vi "LoadDocument__slk_msxml.vi"(0 "document in":refnum<class "msxml document.lvclass">, 1 "xml document path in":path, 11 "error in (no error)":errorcluster, 12 "validate on parse (F)":bool) -> (4 "document out":refnum<class "msxml document.lvclass">, 15 "error out":errorcluster)   [LabVIEW 2020, in "MSXML.lvlib" / "msxml document.lvclass"]
doc: "Loads an XML file to MSXML Document object and allows you to configure the XML parser to validate the file against a schema or DTD (Document Type Definition)."
uses:
  msxml document.lvclass
  msxml document.lvclass/msxml document.ctl
panel:
  # "LoadDocument__slk_msxml.vi\n\nLoads an XML file to MSXML Document object and allows you to configure the XML parser to validate the file against a schema or DTD (Document Type Definition).\n\nNOTICE -- YOU MUST LEAVE THIS NOTICE IN PLACE.\n\nCopyright (c) 2004-2010 Shawn Liu <shawn.liu.cn@gmail.com>\n\nAll rights reserved."
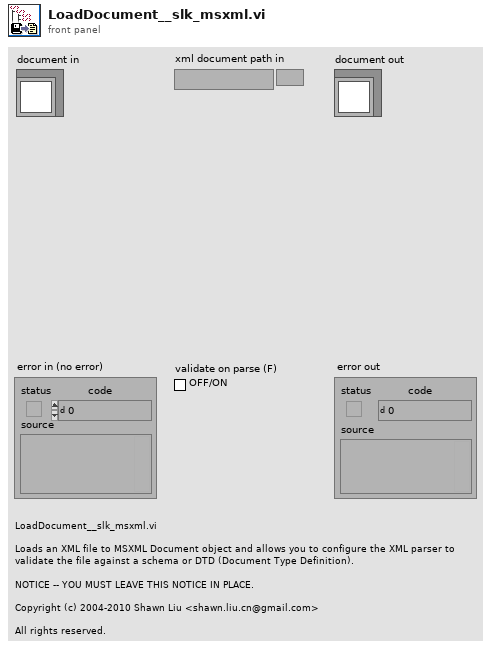
[diagram p1: front panel]
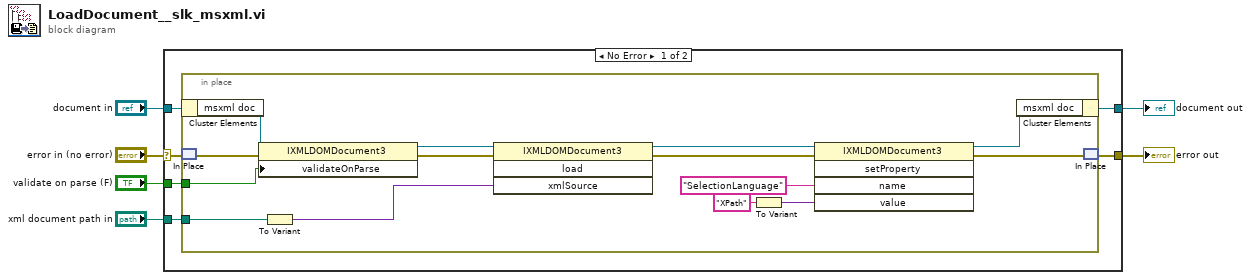
[diagram p0: block diagram]
diagram:
  n1 = case shown="No Error" "error in (no error)" {
    selector: "error in (no error)" -> [w9 w28]
    tunnel: [w8 w28] -> w3
    tunnel: [w7 w27] -> w5
    tunnel: "document in" -> [w10 w27]
    tunnel: "validate on parse (F)" -> [w12 _]
    tunnel: "xml document path in" -> [w11 _]
    frame No Error {
      n2 = in-place {
        in-place-border: w12 -> [w18]
        in-place-border: w11 -> [w17]
        n3 = in-place-cluster #1(w10) -> ("msxml doc"=w16:refnum<k7>)
        n4 = in-place-match #2(w9) -> (w14:errorcluster)
        n5 = property on="Property Node" class="IXMLDOMDocument3"(reference=w16, error in=w14, "validateOnParse"=w18) -> (reference out=w19:refnum<k7>, error out=w20:errorcluster)
        n6 = To Variant(anything=w17) -> (Variant=w24:variant)
        n7 = invoke on="Invoke Node" class="IXMLDOMDocument3" method="load"(reference=w19, error in=w20, "xmlSource"=w24) -> (reference out=w26:refnum<k7>, error out=w25:errorcluster)  [unwired: 1 in, 2 out]
        n8 = To Variant(anything="XPath") -> (Variant=w21:variant)
        n9 = invoke on="Invoke Node" class="IXMLDOMDocument3" method="setProperty"(reference=w26, error in=w25, "name"="SelectionLanguage", "value"=w21) -> (reference out=w15:refnum<k7>, error out=w13:errorcluster)  [unwired: 1 in, 3 out]
        n10 = in-place-cluster #1("msxml doc"=w15) -> (w7:refnum<class "msxml document.lvclass">)
        n11 = in-place-match #2(w13) -> (w8:errorcluster)
      }
    }
    frame Error {
    }
  }
  "document out" <- w5
  "error out" <- w3
